vi "Volt Reader Trigger4.vi"() -> ()   [LabVIEW 2014]
uses:
  <vilib>/Utility/error.llb/DialogType.ctl
  <vilib>/_DAQmxBase/Internals/DAQmxBase Create Channel (AI-Voltage-Basic).vi
  <vilib>/_DAQmxBase/Internals/DAQmxBase Timing (Sample Clock).vi
  <vilib>/_DAQmxBase/Internals/DAQmxBase Read (Analog 2D DBL NChan NSamp).vi
panel:
  in  "Knob":dbl(knob) scale=0.0..10.0
  out "Waveform Graph":waveform(dbl)(graph)
  in  "Buffer (ms)":dbl
  out "Threshold":dbl
  in  "units":i32(ring)=10348 items=["Volts"=10348, "From Custom Scale"=10065]
  in  "stop":bool
  in  "physical channels":tag
  in  "maximum value":dbl=5.0 format="%0.2f"
  in  "minimum value":dbl=-5.0 format="%0.2f"
  in  "rate":i32=1000 caption="Sample Rate"
  # "NOTE: Just change the Y axis value"
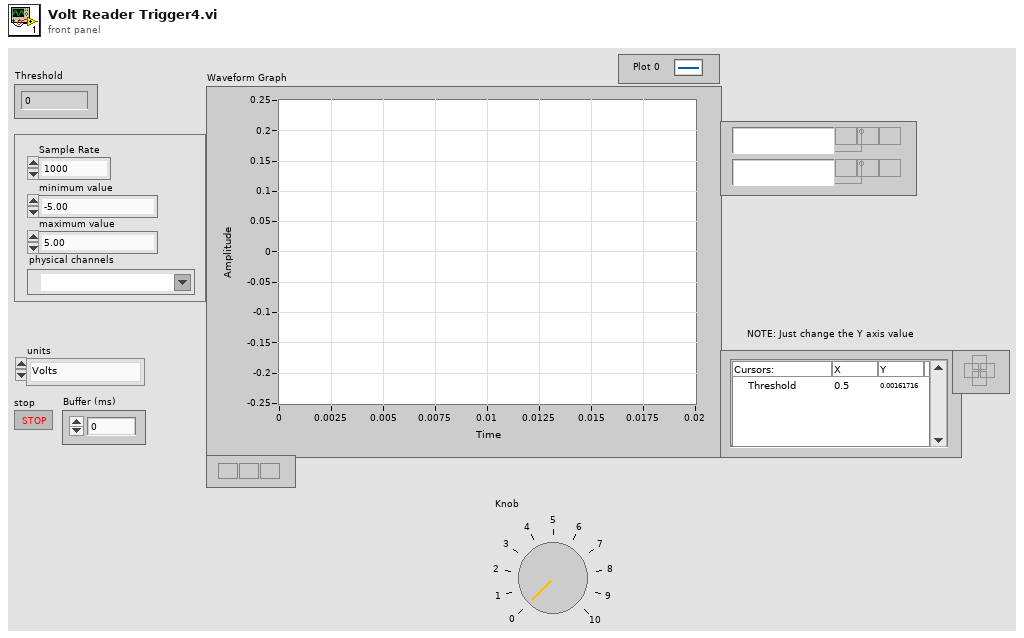
[diagram p1: front panel]
types:
  T1 = typedef "DialogType.ctl" = u16
  T2 = typedef "LVCursorListTypeDef.ctl" = cluster{"Name":string, "Color":u32, "Style":u8, "Point Style":u8, "Name Visible":bool, "Allow Drag":bool, "Cursor Mode":u32, "Plot":i32, "Index":i32, "Position":cluster{"X":dbl, "Y":dbl}, "X Scale":u32, "Y Scale":u32, "Watch Plots":i32[], "Watch All Plots":bool, "Plot Area":i32, "Label Offset":cluster{"X":dbl, "Y":dbl}}[]
  T3 = cluster{"Name":string, "Color":u32, "Style":u8, "Point Style":u8, "Name Visible":bool, "Allow Drag":bool, "Cursor Mode":u32, "Plot":i32, "Index":i32, "Position":cluster{"X":dbl, "Y":dbl}, "X Scale":u32, "Y Scale":u32, "Watch Plots":i32[], "Watch All Plots":bool, "Plot Area":i32, "Label Offset":cluster{"X":dbl, "Y":dbl}}
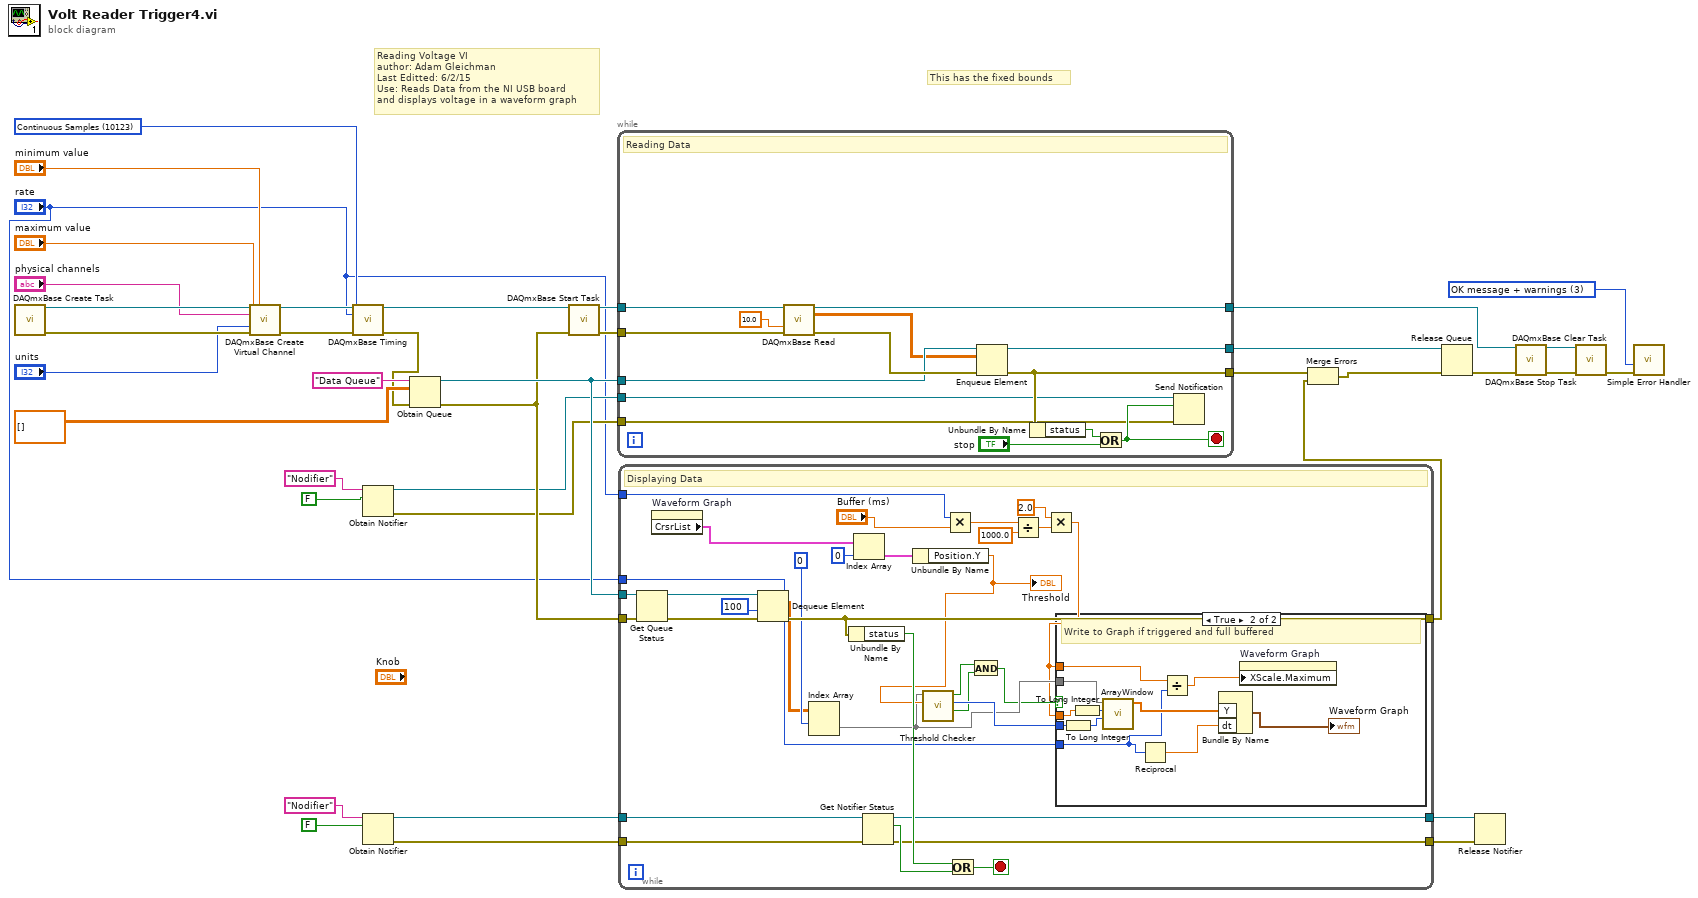
[diagram p0: block diagram]
diagram:
  w15 = 10123 items=["Finite Samples"=10178, "Continuous Samples"=10123, "Hardware Timed Single Point"=12522] ("sample mode")
  w17 = T1 3 items=["no dialog", "OK message", "continue or stop message", "OK message + warnings", "continue/stop + warnings"] ("type of dialog (OK msg:1)")
  # "This has the fixed bounds"
  # "Reading Voltage VI\nauthor: Adam Gleichman\nLast Editted: 6/2/15 \nUse: Reads Data from the NI USB board\nand displays voltage in a waveform graph"
  n1 = call <vilib>:"DAQmxBase Create Task.vi"() -> ("task out"=w37:refnum<k21>, "error out"=w36:errorcluster)  [unwired: 5 in, 9 out]
  n2 = call-poly <vilib>:"DAQmxBase Create Virtual Channel.vi"("task in"=w37, "maximum value"="maximum value", "minimum value"="minimum value", "physical channels"="physical channels", "units"="units", "error in"=w36) -> ("task out"=w34:refnum<k21>, "error out"=w35:errorcluster)  [unwired: 3 in, 5 out]
  n3 = call-poly <vilib>:"DAQmxBase Timing.vi"("task/channels in"=w34, "sample mode"=w15, "rate"="rate", "error in"=w35) -> ("task out"=w3:refnum<k21>, "error out"=w2:errorcluster)  [unwired: 3 in, 7 out]
  n4 = Obtain Notifier(name (unnamed)="Nodifier", notification data type=FALSE) -> (notifier out=w11:refnum<notifier>, error out=w10:errorcluster)  [unwired: 2 in, 1 out]
  n5 = Obtain Notifier(name (unnamed)="Nodifier", notification data type=FALSE) -> (notifier out=w8:refnum<notifier>, error out=w6:errorcluster)  [unwired: 2 in, 1 out]
  n6 = Obtain Queue(name (unnamed)="Data Queue", element data type=dbl[][] [] ("data"), error in (no error)=w2) -> (queue out=w24:refnum<queue>, error out=w23:errorcluster)  [unwired: 2 in, 1 out]
  n7 = call <vilib>:"DAQmxBase Start Task.vi"("task/channels in"=w3, "error in"=w23) -> ("task out"=w32:refnum<k21>, "error out"=w33:errorcluster)  [unwired: 12 out]
  n8 = while "Data Reading Loop" {
    tunnel: w33 -> [w51]
    tunnel: w32 -> [w52]
    tunnel: w24 -> [w49]
    tunnel: [w46] -> w27
    tunnel: [w44] -> w26
    tunnel: [w42] -> w14
    tunnel: w11 -> [w40]
    tunnel: w10 -> [w39]
    stop <- w41 stop-if-true
    # "Reading Data"
    n9 = call-poly <vilib>:"DAQmxBase Read.vi"("task/channels in"=w52, "timeout"=10.0, "error in"=w51) -> ("task out"=w42:refnum<k21>, "data"=w47:dbl[][], "error out"=w50:errorcluster)  [unwired: 10 in]
    n10 = Enqueue Element(queue=w49, element=w47, error in (no error)=w50) -> (queue out=w46:refnum<queue>, error out=w44:errorcluster)  [unwired: 1 in, 1 out]
    n11 = Unbundle By Name(w44) -> ("status"=w43:bool)
    n12 = Or(x=w43, y="stop") -> (x .or. y?=w41:bool)
    n13 = Send Notification(notification=w41, notifier=w40, error in (no error)=w39) -> ()  [unwired: 2 out]
  }
  n14 = while {
    tunnel: w24 -> [w84]
    tunnel: w23 -> [w73]
    tunnel: [w82] -> w22
    tunnel: w8 -> [w79]
    tunnel: w6 -> [w78]
    tunnel: [w76] -> w4
    tunnel: [w75] -> w5
    tunnel: "rate" -> [w68]
    tunnel: "rate" -> [w61]
    stop <- w80 stop-if-true
    # "Displaying Data"
    n15 = Get Queue Status(queue=w84, error in (no error)=w73) -> (queue out=w74:refnum<queue>, error out=w72:errorcluster)  [unwired: 1 in, 6 out]
    n16 = property on="Waveform Graph" class="WFGraph (strict)"() -> ("CrsrList"=w66:T2)  [unwired: 2 in, 2 out]
    n17 = Dequeue Element(queue=w74, timeout in ms (-1)=100, error in (no error)=w72) -> (element=w70:dbl[][], error out=w82:errorcluster)  [unwired: 2 out]
    n18 = Index Array(array=w70, index (row)=0 ("index")) -> (element=w55:dbl[])  [unwired: 1 in]
    n19 = Unbundle By Name(w82) -> ("status"=w81:bool)
    n20 = Index Array(array=w66, index=0) -> (element=w65:T3)
    n21 = Get Notifier Status(notifier=w79, error in (no error)=w78) -> (notifier out=w76:refnum<notifier>, current notification=w77:bool, error out=w75:errorcluster)  [unwired: 2 out]
    n22 = Unbundle By Name(w65) -> ("Position.Y"=w64:dbl)
    "Threshold" <- w64
    n23 = call "Threshold Checker.vi"("Threshold"=w64, "Data"=w55) -> ("buffer filled?"=w56:bool, "Index of Value = to or exceeding threshold"=w69:i32, "Did we pass the threshold?"=w57:bool)  [unwired: 7 in]
    n24 = Multiply(x=w61, y="Buffer (ms)") -> (x*y=w63:dbl)
    n25 = Or(x=w81, y=w77) -> (x .or. y?=w80:bool)
    n26 = And(x=w57, y=w56) -> (x .and. y?=w54:bool)
    n27 = Divide(x=w63, y=1000.0) -> (x/y=w60:dbl)
    n28 = Multiply(x=2.0, y=w60) -> (x*y=w53:dbl)
    n29 = case shown="True" w54 {
      tunnel: w53 -> [_ w92]
      tunnel: w69 -> [_ w91]
      tunnel: w68 -> [_ w86]
      tunnel: w55 -> [_ w88]
      tunnel: w53 -> [_ w87]
      frame False {
        # "Write nothing on the graph"
      }
      frame True {
        # "Write to Graph if triggered and full buffered"
        n30 = To Long Integer(number=w91) -> (32bit integer=w90:i32)
        n31 = To Long Integer(number=w92) -> (32bit integer=w89:i32)
        n32 = call "ArrayWindow.VI"("Index"=w90, "Total amount of Pts"=w89, "Input Y-values"=w88) -> ("Output Array"=w93:dbl[])  [unwired: 8 in]
        n33 = Reciprocal(x=w86) -> (1/x=w95:dbl)
        n34 = Divide(x=w87, y=w86) -> (x/y=w85:dbl)
        n35 = Bundle By Name("Y"=w93, "dt"=w95) -> (→"Waveform Graph":waveform(dbl))  [unwired: 1 in]
        n36 = property on="Waveform Graph" class="WFGraph (strict)"("XScale.Maximum"=w85) -> ()  [unwired: 2 in, 2 out]
      }
    }
  }
  n37 = Merge Errors(w26, w22) -> (w25:errorcluster)
  n38 = Release Queue(queue=w27, error in (no error)=w25) -> (error out=w21:errorcluster)  [unwired: 1 in, 2 out]
  n39 = Release Notifier(notifier=w4, error in (no error)=w5) -> ()  [unwired: 1 in, 3 out]
  n40 = call <vilib>:"DAQmxBase Stop Task.vi"("task/channels in"=w14, "error in"=w21) -> ("task out"=w20:refnum<k21>, "error out"=w19:errorcluster)  [unwired: 12 in]
  n41 = call <vilib>:"DAQmxBase Clear Task.vi"("task in"=w20, "error in"=w19) -> ("error out"=w18:errorcluster)  [unwired: 13 in]
  n42 = call <vilib>:"Simple Error Handler.vi"("type of dialog (OK msg:1)"=w17, "error in (no error)"=w18) -> ()  [unwired: 3 in, 5 out]
